vi "MyProject.vi"() -> ()   [LabVIEW 2018]
panel:
  out "?":bool
  out "Sensor Value":i32
  out "Chart":i32(graph)
  out "error DataBase":errorcluster
  out "error VISA":errorcluster
  in  "?":bool
  in  "?":bool
  in  "Utilisateur":string
  in  "Mot de passe":string
  in  "VISA  in":refnum<visa-resource-name>
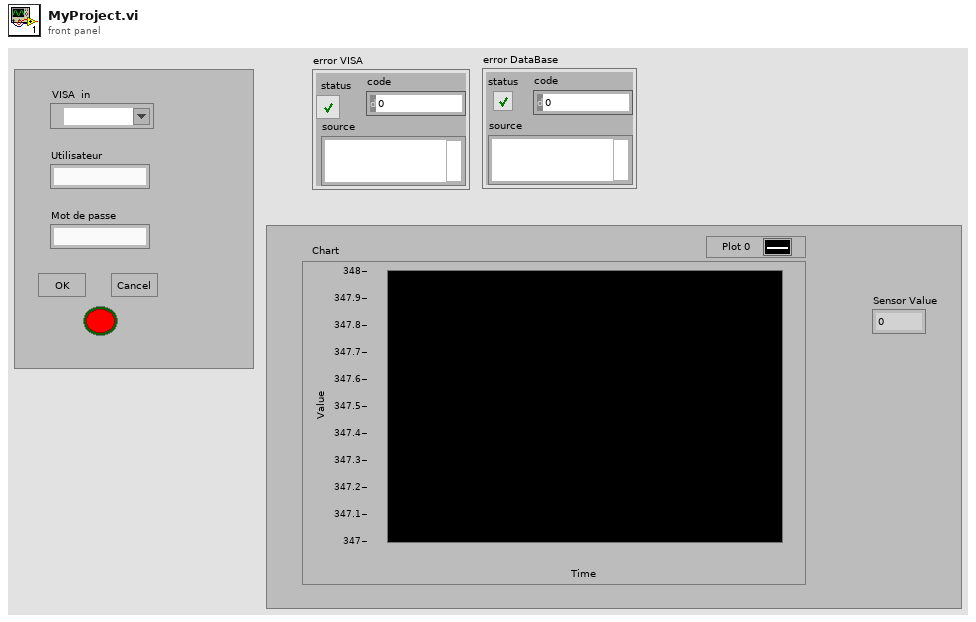
[diagram p1: front panel]
types:
  T1 = typedef "NI_Database_API.lvlib/Conn ObjectReference.ctl" = refnum<k1>
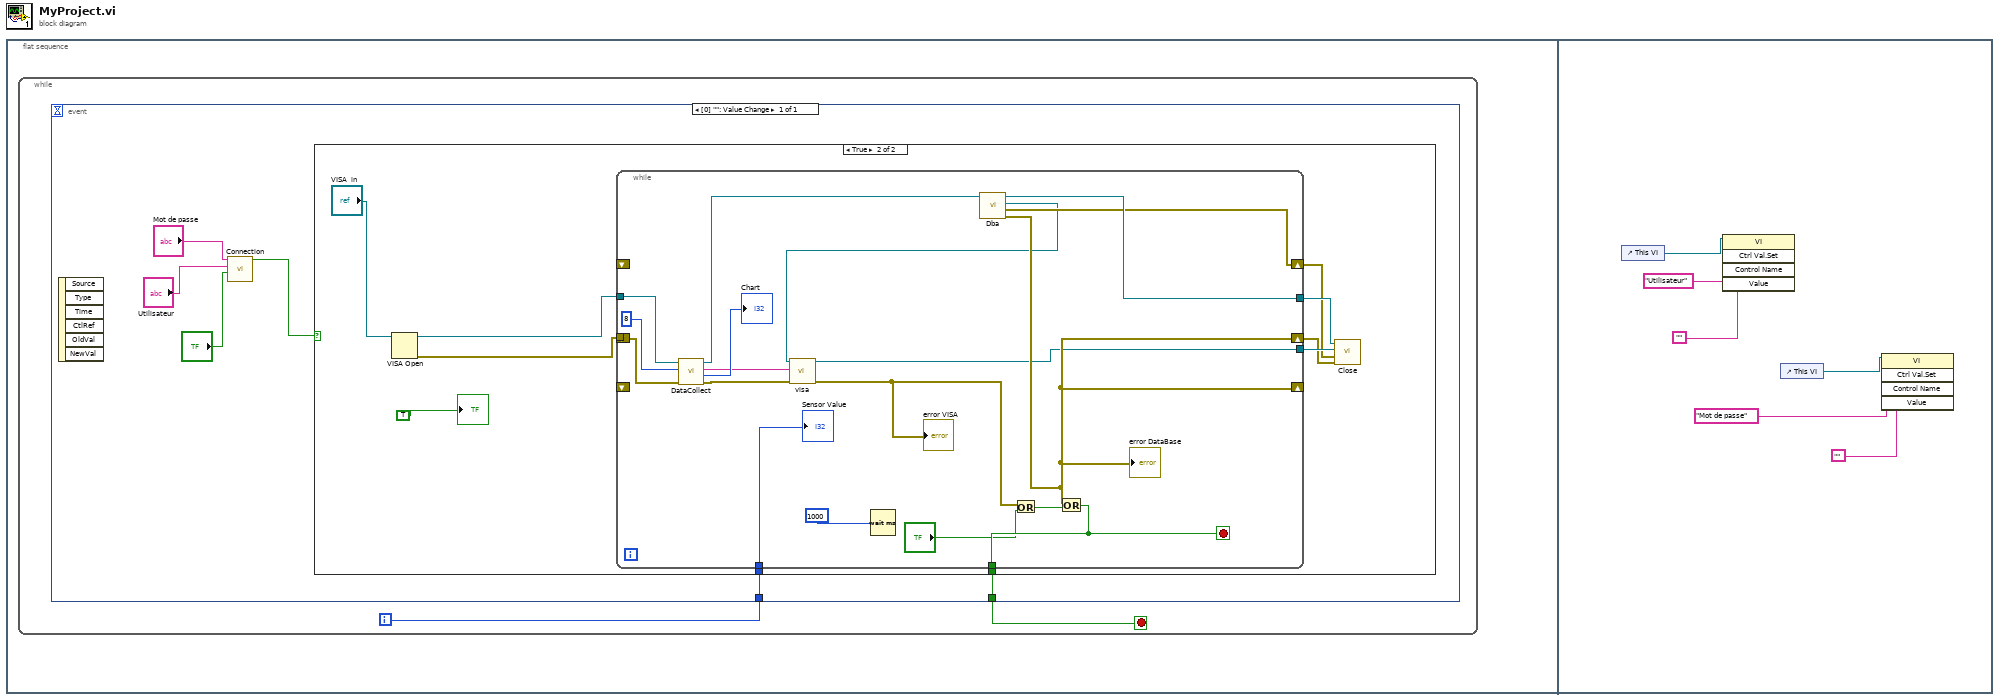
[diagram p0: block diagram]
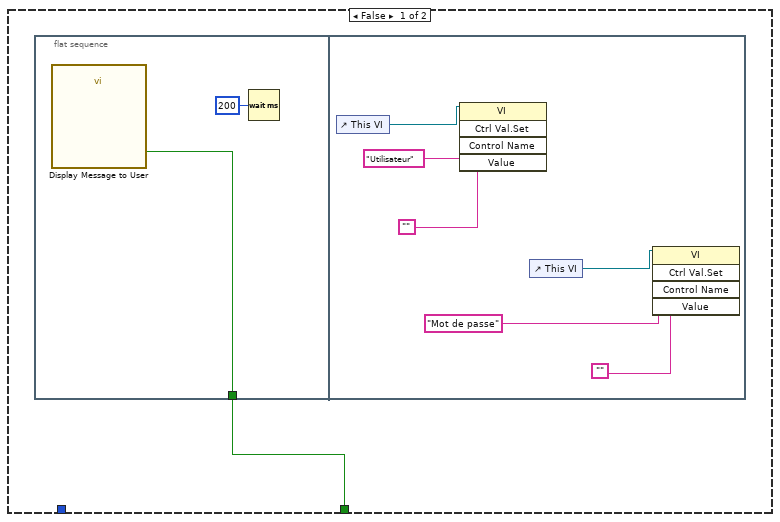
[diagram p2: hidden frame]
diagram:
  n1 = flat-sequence {
    frame #0 {
      n2 = while {
        i -> [w1]
        stop <- w2 stop-if-true
        n3 = event shown="[0] \"\": Value Change" {
          selector: _ -> [_]
          dyn-events: _ -> [_]
          timeout: _ -> [_]
          tunnel: [w8] -> w2
          tunnel: w1 -> [w3]
          event Value Change {
            n4 = event-data() -> ()  [unwired: 1 in, 6 out]
            n5 = call "Connection.vi"(9:"?", "Utilisateur"="Utilisateur", "Mot_de_passe"="Mot de passe") -> ("Boolean"=w4:bool)  [unwired: 8 in]
            n6 = case shown="True" w4 {
              tunnel: [w9 w27] -> w8
              tunnel: w3 -> [_ w22]
              frame False {
                n7 = flat-sequence {
                  tunnel: [w11] -> w9
                  frame #0 {
                    n8 = call "Display Message to User"() -> ("OK"=w11:bool)  [unwired: 10 in, 1 out]
                    n9 = Wait (ms)(milliseconds to wait=u32 200) -> ()  [unwired: 1 out]
                  }
                  frame #1 {
                    n10 = control-ref of="This VI"() -> (w13:refnum<vi>)
                    n11 = invoke class="VI" method="Ctrl Val.Set"(reference=w13, "Control Name"="Utilisateur", "Value"="") -> ()  [unwired: 2 in, 5 out]
                    n12 = control-ref of="This VI"() -> (w16:refnum<vi>)
                    n13 = invoke class="VI" method="Ctrl Val.Set"(reference=w16, "Control Name"="Mot de passe", "Value"="") -> ()  [unwired: 2 in, 5 out]
                  }
                }
              }
              frame True {
                n14 = VISA Open(VISA resource name="VISA  in") -> (VISA resource name=w24:refnum<visa-resource-name>, error out=w23:errorcluster)  [unwired: 4 in]
                n15 = while {
                  tunnel: [w45] -> w20
                  shift-right: [w42] -> w19
                  shift-left: _ -> [w37]
                  shift-right: [w31] -> w18
                  shift-left: _ -> [_]
                  shift-right: [w42] -> _
                  shift-left: _ -> [_]
                  tunnel: [w41] -> w27
                  tunnel: w24 -> [w39]
                  tunnel: w23 -> [_]
                  tunnel: w22 -> [w34]
                  tunnel: [w32] -> w21
                  stop <- w41 stop-if-true
                  n16 = call "DataCollect.vi"("error in (no error)"=w37, "byte count"=u32 8, "VISA Refnum in"=w39) -> ("error out"=w30:errorcluster, "Numeric"=→"Chart":i32, "read buffer"=w29:string, "VISA Refnum out"=w36:refnum<visa-resource-name>)  [unwired: 5 in]
                  n17 = Wait (ms)(milliseconds to wait=u32 1000) -> ()  [unwired: 1 out]
                  n18 = call "Dba.vi"("VISA Refnum in"=w36) -> (0:"error out"=w42:errorcluster, 1:"error out"=w31:errorcluster, "connection reference"=w28:T1, "VISA Refnum out"=w45:refnum<visa-resource-name>)  [unwired: 7 in]
                  "error DataBase" <- w42
                  n19 = call "visa.vi"("error in (no error)"=w30, "read buffer"=w29, "Refnum in"=w28) -> ("error out"=w35:errorcluster, "Refnum out"=w32:T1)  [unwired: 7 in]
                  "error VISA" <- w35
                  n20 = Or(x=w35, y="?") -> (x .or. y?=w44:bool)
                  n21 = Or(x=w42, y=w44) -> (x .or. y?=w41:bool)
                  "Sensor Value" <- w34
                }
                n22 = call "Close.vi"("error in (no error)"=w19, "error in"=w18, "Refnum in"=w21, "VISA Refnum in"=w20) -> ()  [unwired: 8 in]
                "?" <- TRUE
              }
            }
          }
        }
      }
    }
    frame #1 {
      n23 = control-ref of="This VI"() -> (w51:refnum<vi>)
      n24 = invoke class="VI" method="Ctrl Val.Set"(reference=w51, "Control Name"="Utilisateur", "Value"="") -> ()  [unwired: 2 in, 5 out]
      n25 = control-ref of="This VI"() -> (w48:refnum<vi>)
      n26 = invoke class="VI" method="Ctrl Val.Set"(reference=w48, "Control Name"="Mot de passe", "Value"="") -> ()  [unwired: 2 in, 5 out]
    }
  }
